vi "AddCORSHeaders.vi"(8 "error in (no error)":errorcluster, 11 "LabVIEW Web Service Request":refnum<class "Web Request.lvclass">) -> (0 "error out":errorcluster, 3 "LabVIEW Web Service Request out":refnum<class "Web Request.lvclass">)   [LabVIEW 2019]
uses:
  <vilib>/wsapi/Web Request.lvclass
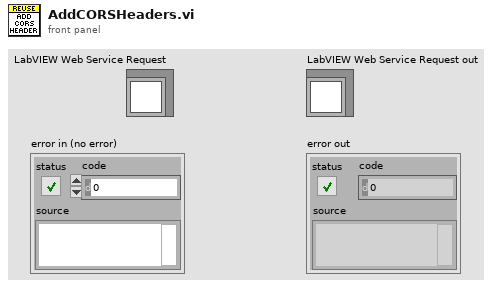
[diagram p1: front panel]
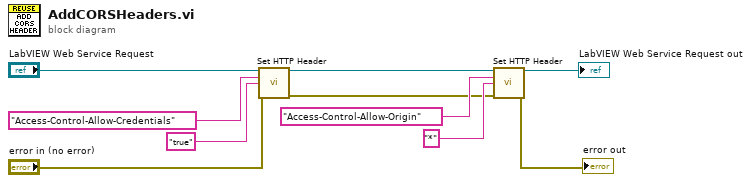
[diagram p0: block diagram]
diagram:
  n1 = call <vilib>:"Set HTTP Header.vi"("LabVIEW Web Service Request"="LabVIEW Web Service Request", "header"="Access-Control-Allow-Credentials", "header value"="true" ("header"), "error in (no error)"="error in (no error)") -> ("LabVIEW Web Service Request out"=w5:refnum<class "Web Request.lvclass">, "error out"=w3:errorcluster)  [unwired: 10 in]
  n2 = call <vilib>:"Set HTTP Header.vi"("LabVIEW Web Service Request"=w5, "header"="Access-Control-Allow-Origin", "header value"="*" ("header"), "error in (no error)"=w3) -> ("LabVIEW Web Service Request out"=→"LabVIEW Web Service Request out":refnum<class "Web Request.lvclass">, "error out"=→"error out":errorcluster)  [unwired: 10 in]
